vi "Vision Processing.vi"(4 "error in (no error)":errorcluster, 6 "CameraDevRef":T1) -> ()   [LabVIEW 2011]
uses:
  <vilib>/Rock Robotics/WPI/Camera/WPI_CameraDevRef.ctl
  Robot Global Data.vi
  <vilib>/vision/NI_Vision_Development_Module.lvlib
panel:
  out "Aspect Ratio":dbl[](array[numeric])
  out "Offset":dbl
  in  "Max Distance for 1 hoop":dbl=8.0
  out "Raw Turret":dbl
  in  "Run Calculations":bool
  out "Target X Coord":dbl
  out "Target Distance":dbl
  out "Target Y Coord":dbl
  out "Distance Array":dbl[](array[numeric])
  in  "Scaler":dbl=0.85
  in  "Dead Band":dbl=0.05
  out "Number of Rectangles Visible":dbl
  out "Y Position Array":dbl[](array[numeric])
  out "X Position Array":dbl[](array[numeric])
  in  "View":bool
  out "Target Info":T2(array[cluster])
  in  "Area Size Limit":i32=444
  in  "Particle Count Limit":i32=8
  in  "Score Limits":T3={"Rect Coverage"=76.0, "Aspect Ratio"=40.0, "X Edge Strength"=40.0, "Y Edge Strength"=60.0}
  in  "Processing":enum32{"Color", "Intensity", "Intensity Open"}(tab)=enum."Intensity"
  in  "Luminance":i32=255
  in  "Saturation":i32=255
  in  "Hue":i32(knob)=65 scale=0.0..255.0
  in  "Margins":cluster{"Hue":i32, "Sat":i32, "Lum":i32}={"Hue"=20, "Sat"=27, "Lum"=30} {"Sat" scale=0.0..40.0; "Lum" scale=0.0..40.0; "Hue" scale=0.0..40.0}
  in  "Range":cluster{"Lower value":sgl, "Upper value":sgl}={"Lower value"=107.17391, "Upper value"=255.0} {"Lower value" scale=0.0..255.0; "Upper value" scale=0.0..255.0}
  in  "Range":cluster{"Lower value":sgl, "Upper value":sgl}={"Lower value"=123.804344, "Upper value"=255.0} {"Lower value" scale=0.0..255.0; "Upper value" scale=0.0..255.0}
  in  "View":bool
  out "Processed Image":T4(plugin-control)
  out "Original Image":T4(plugin-control)
  # "Instructions:\nProcessing the reflective tape that is illuminated by a ring light can be based\non color or light intensity.\nParticles within the image are scored by rectangle coverage, aspect ratio, and\nfor being hollow with a bold edge. A particle is considered a target if all scores\nare above the score limits. Particles can be annotated -- surrounded by\na rectangle and scores drawn to the left .\nTo control the number of particles being scored, use the count limit and the size\nlimit."
  # "(in)"
  # "To debug, Enable using the View button.\nFor color processing, you can click in the image to select the color for processing."
  # "Enable by clicking the View button.\nGreen scores are above the limit, orange are below. Inner/outer rect\nindicates all passed."
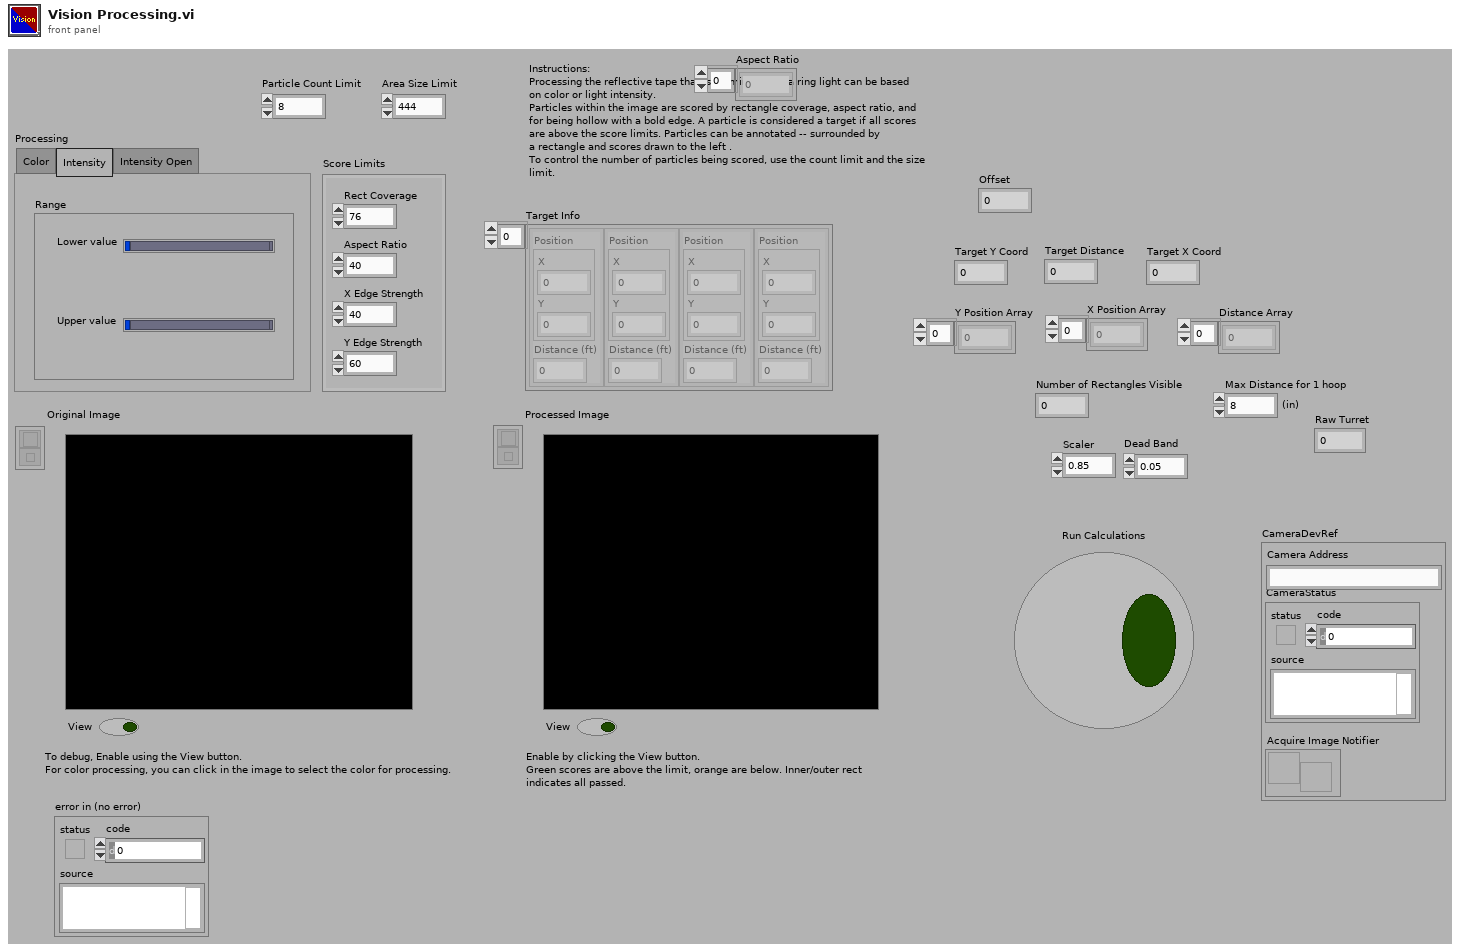
[diagram p1: front panel]
types:
  T1 = typedef "WPI_CameraDevRef.ctl" = cluster{"Camera Address":string, "CameraStatus":errorcluster, "Acquire Image Notifier":refnum<notifier>}
  T2 = cluster{"Position":cluster{"X":dbl, "Y":dbl}, "Distance (ft)":dbl}[]
  T3 = cluster{"Rect Coverage":dbl, "Aspect Ratio":dbl, "X Edge Strength":dbl, "Y Edge Strength":dbl}
  T4 = typedef "IMAQ Image.ctl" = refnum<image>
  T5 = typedef "Image Type" = u32
  T6 = enum32{"AutoM", "Close", "Dilate", "Erode", "Gradient", "Gradient out", "Gradient in", "Hit miss", "Open", "PClose", "POpen", "Thick", "Thin"}
  T7 = typedef "WPI_CameraImageSize.ctl" = enum16{"640x480", "320x240", "160x120"}
  T8 = cluster{"fps":i32, "compression":i32, "Image Size":T7}
  T9 = cluster{cluster{"Left":dbl, "Top":dbl, "Right":dbl, "Bottom":dbl}, dbl[]}[]
  T10 = cluster{"Left":dbl, "Top":dbl, "Right":dbl, "Bottom":dbl}
  T11 = cluster{"Target Center (-1 to 1)":cluster{"X":dbl, "Y":dbl}, "Distance (ft)":dbl}
  T12 = cluster{"Target Center (-1 to 1)":cluster{"X":dbl, "Y":dbl}, "Distance (ft)":dbl}[]
  T13 = typedef "WPI_JoystickDevRef.ctl" = cluster{"Device":T14}
  T14 = typedef "WPI_JoystickDeviceEnum.ctl" = enum16{"USB 1", "USB 2", "USB 3", "USB 4", "Kinect 1", "Kinect 2"}
  T15 = typedef "WPI_JoystickButtonState.ctl" = cluster{"Button 1":bool, "Button 2":bool, "Button 3":bool, "Button 4":bool, "Button 5":bool, "Button 6":bool, "Button 7":bool, "Button 8":bool, "Button 9":bool, "Button 10":bool, "Button 11":bool, "Button 12":bool}
  T16 = cluster{"axis 1 (x)":dbl, "axis 2 (y)":dbl, "axis 3 (throttle)":dbl, "axis 4":dbl, "axis 5":dbl, "axis 6":dbl}
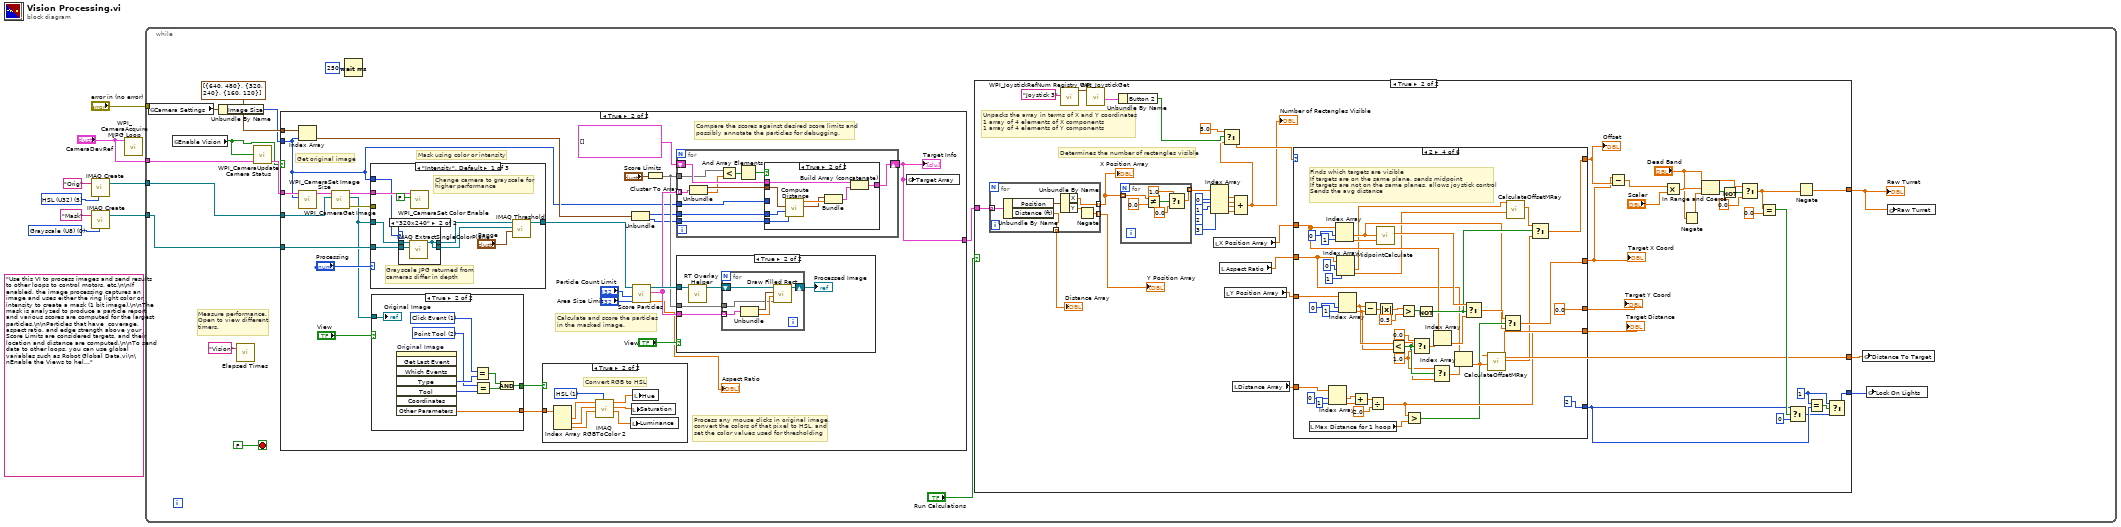
[diagram p0: block diagram]
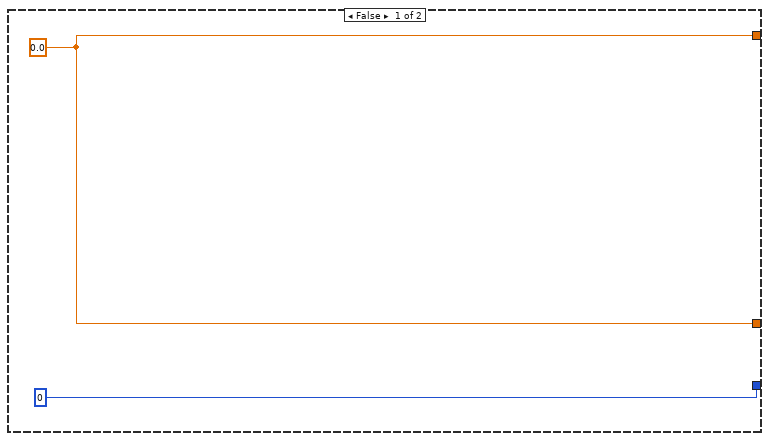
[diagram p2: hidden frame]
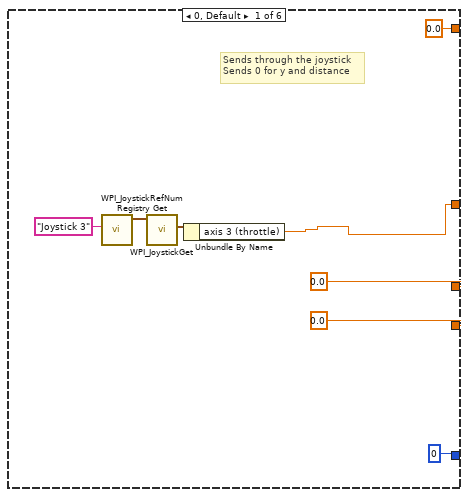
[diagram p3: hidden frame]
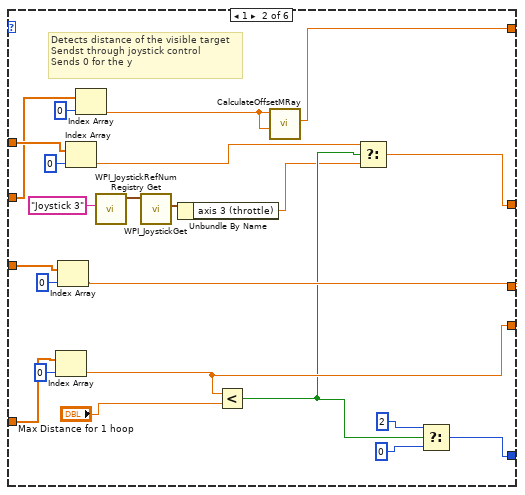
[diagram p4: hidden frame]
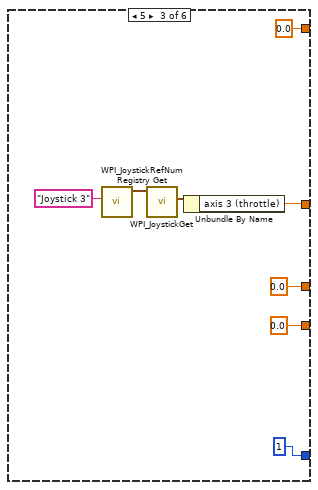
[diagram p5: hidden frame]
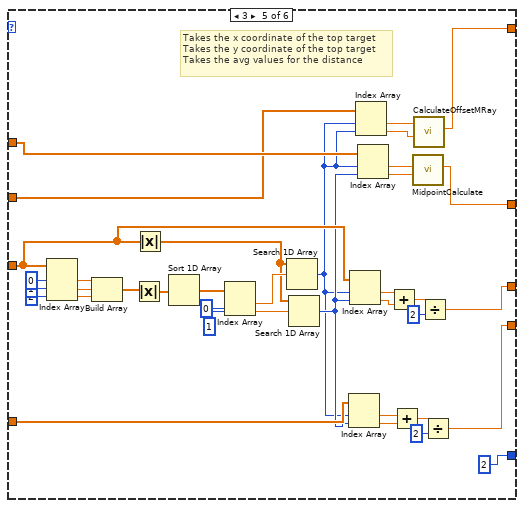
[diagram p6: hidden frame]
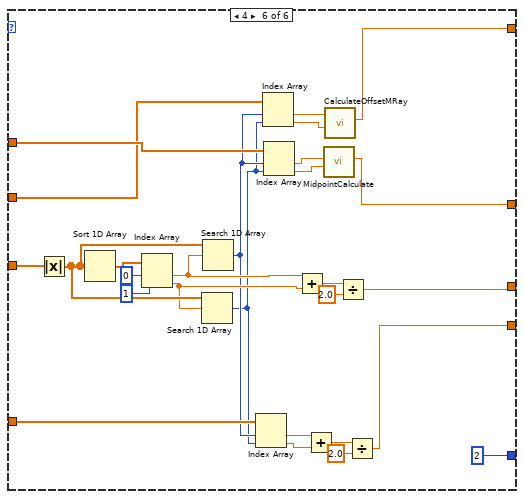
[diagram p7: hidden frame]
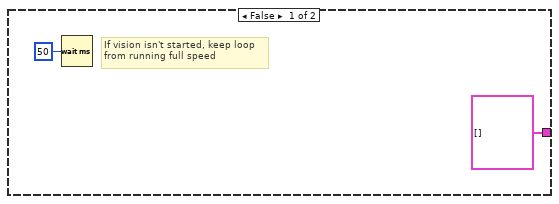
[diagram p8: hidden frame]
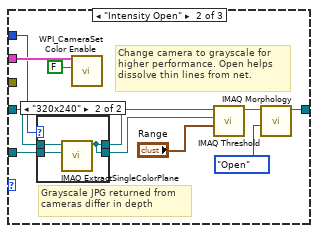
[diagram p11: hidden frame]
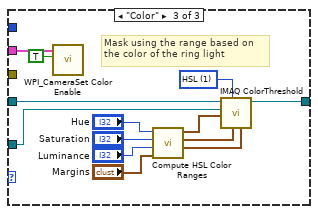
[diagram p13: hidden frame]
diagram:
  w3 = T5 0 items=["Grayscale (U8)", "Grayscale (I16)", "Grayscale (SGL)", "Complex (CSG)", "RGB (U32)", "HSL (U32)", "RGB (U64)", "Grayscale (U16)"] ("Image Type")
  (unwired) "Use this VI to process images and send results to other loops to control motors, etc.\n\nIf enabled, the image processing captures an image and uses either the ring light color or intensity to create a mask (1 bit image).\n\nThe mask is analyzed to produce a particle report and various scores are computed for the largest particles.\n\nParticles that have  coverage, aspect ratio, and edge strength above your Score Limits are considered targets, and their location and distance are computed.\n\nTo send data to other loops, you can use global variables such as Robot Global Data.vi\n\nEnable the Views to help debug color settings. Disable the View to speed up processing."
  w7 = T5 5 items=["Grayscale (U8)", "Grayscale (I16)", "Grayscale (SGL)", "Complex (CSG)", "RGB (U32)", "HSL (U32)", "RGB (U64)", "Grayscale (U16)"] ("Image Type")
  n1 = call "IMAQ Create"("Image Name"="Orig", "Image Type"=w7) -> ("New Image"=w6:T4)  [unwired: 2 in, 2 out]
  n2 = call "IMAQ Create"("Image Name"="Mask", "Image Type"=w3) -> ("New Image"=w1:T4)  [unwired: 2 in, 2 out]
  n3 = call <vilib>:"WPI_CameraAcquire MJPG Loop.vi"("CameraDevRef"="CameraDevRef") -> ()  [unwired: 11 in]
  n4 = while {
    tunnel: w6 -> [w23]
    tunnel: "CameraDevRef" -> [w22]
    tunnel: "error in (no error)" -> [_]
    tunnel: w1 -> [w18]
    stop <- FALSE stop-if-true
    # "Measure performance.\nOpen to view different\ntimers."
    n5 = global read "Robot Global Data.vi" "Camera Settings"() -> (w16:T8)
    n6 = global read "Robot Global Data.vi" "Enable Vision"() -> (w20:bool)
    n7 = Unbundle By Name(w16) -> ("Image Size"=w15:T7)
    n8 = call "Elapsed Times.vi"("Call Name"="Vision") -> ()  [unwired: 2 in, 1 out]
    n9 = call <vilib>:"WPI_CameraUpdate Camera Status.vi"("CameraDevRef In"=w22, "Enable Vision"=w20) -> ("CameraDevRef Out"=w21:T1)  [unwired: 3 in]
    n10 = case shown="True" w20 {
      tunnel: w23 -> [_ w252]
      tunnel: w21 -> [_ w248]
      tunnel: w18 -> [_ w239]
      tunnel: cluster{i32, i32}[] [{640, 480}, {320, 240}, {160, 120}] -> [_ w243]
      tunnel: w15 -> [_ w236]
      tunnel: [T2 [] w237] -> w14
      frame False {
        # "If vision isn't started, keep loop\nfrom running full speed"
        n11 = Wait (ms)(milliseconds to wait=u32 50) -> ()  [unwired: 1 out]
      }
      frame True {
        # "Compare the scores against desired score limits and\npossibly annotate the particles for debugging."
        # "Process any mouse clicks in original image,\nconvert the colors of that pixel to HSL, and\nset the color values used for thresholding"
        # "Calculate and score the particles\nin the masked image."
        # "Mask using color or intensity"
        # "Get original image"
        n12 = call <vilib>:"WPI_CameraSet Image Size.vi"("Image Size"=w236, "CameraDevRef"=w248) -> ("CameraDevRef Out"=w249:T1)  [unwired: 8 in, 1 out]
        n13 = Index Array(array=w243, index=w236) -> (element=w240:cluster{i32, i32})
        n14 = call <vilib>:"WPI_CameraGet Image.vi"("Image"=w252, "CameraDevRef"=w249) -> ("error out"=w250:errorcluster, "Image Out"=w238:T4, "CameraDevRef Out"=w251:T1)  [unwired: 7 in]
        n15 = case shown="\"Intensity\", Default" "Processing" {
          tunnel: w238 -> [w274 w286 w312]
          tunnel: [w277 w291 w311] -> w246
          tunnel: w251 -> [w275 w289 w302]
          tunnel: w250 -> [_ _ _]
          tunnel: w239 -> [w273 w287 w300]
          tunnel: w236 -> [w272 w288 _]
          frame "Intensity", Default {
            # "Grayscale JPG returned from\ncameras differ in depth"
            # "Change camera to grayscale for\nhigher performance"
            n16 = case shown="\"320x240\"" w272 {
              tunnel: w274 -> [w280 w283]
              tunnel: w273 -> [w279 w282]
              tunnel: [w280 w281] -> w271
              tunnel: [w279 w281] -> w270
              frame "640x480", Default {
              }
              frame "320x240" {
                n17 = call "IMAQ ExtractSingleColorPlane"("Image Dst"=w282, "Image Src"=w283) -> ("Image Dst Out"=w281:T4)  [unwired: 8 in, 1 out]
              }
            }
            n18 = call <vilib>:"WPI_CameraSet Color Enable.vi"("Color Enabled"=FALSE, "CameraDevRef"=w275) -> ()  [unwired: 8 in, 2 out]
            n19 = call "IMAQ Threshold"("Range"="Range", "Image Dst"=w270, "Image Src"=w271) -> ("Image Dst Out"=w277:T4)  [unwired: 3 in, 5 out]
          }
          frame "Intensity Open" {
            # "Grayscale JPG returned from\ncameras differ in depth"
            # "Change camera to grayscale for\nhigher performance. Open helps\ndissolve thin lines from net."
            n20 = case shown="\"320x240\"" w288 {
              tunnel: w286 -> [w296 w299]
              tunnel: w287 -> [w295 w298]
              tunnel: [w296 w297] -> w285
              tunnel: [w295 w297] -> w284
              frame "640x480", Default {
              }
              frame "320x240" {
                n21 = call "IMAQ ExtractSingleColorPlane"("Image Dst"=w298, "Image Src"=w299) -> ("Image Dst Out"=w297:T4)  [unwired: 8 in, 1 out]
              }
            }
            n22 = call <vilib>:"WPI_CameraSet Color Enable.vi"("Color Enabled"=FALSE, "CameraDevRef"=w289) -> ()  [unwired: 8 in, 2 out]
            n23 = call "IMAQ Threshold"("Range"="Range", "Image Dst"=w284, "Image Src"=w285) -> ("Image Dst Out"=w292:T4)  [unwired: 3 in, 5 out]
            n24 = call "IMAQ Morphology"("Operation"=T6."Open", "Image Src"=w292) -> ("Image Dst Out"=w291:T4)  [unwired: 8 in, 1 out]
          }
          frame "Color" {
            w310 = u16 1 items=["RGB", "HSL", "HSV", "HSI"] ("Color Mode")
            # "Mask using the range based on\nthe color of the ring light"
            n25 = call <vilib>:"WPI_CameraSet Color Enable.vi"("Color Enabled"=TRUE, "CameraDevRef"=w302) -> ()  [unwired: 8 in, 2 out]
            n26 = call "Compute HSL Color Ranges.vi"("Margins"="Margins", "Luminance"="Luminance", "Saturation"="Saturation", "Hue"="Hue") -> ("Lum Range"=w307:cluster{i32, i32}, "Sat Range"=w308:cluster{i32, i32}, "Hue Range"=w309:cluster{i32, i32})  [unwired: 5 in]
            n27 = call "IMAQ ColorThreshold"("Blue or Luma or Val or Inten Range"=w307, "Green or Sat Range"=w308, "Color Mode"=w310, "Red or Hue Range"=w309, "Image Dst"=w300, "Image Src"=w312) -> ("Image Dst Out"=w311:T4)  [unwired: 4 in, 1 out]
          }
        }
        n28 = case shown="True" "View" {
          tunnel: w238 -> [_ w332]
          tunnel: [_ w327] -> w245
          tunnel: [_ w324] -> w244
          frame False {
          }
          frame True {
            w325 = 2 items=["None", "Selection Tool", "Point Tool", "Line Tool", "Rectangle Tool", "Oval Tool", "Polygon Tool", "ClosedFreehandTool", "Annulus Tool", "Rotated Rectangle Tool", "Zoom Tool", "Pan Tool", "Polyline Tool", "Freehand Tool"] ("Tool")
            w326 = 1 items=["No Event"=0, "Click Event"=1, "Draw Event"=2, "Size Event"=4, "Scroll Event"=5, "Double Click Event"=8] ("Type")
            n29 = invoke on="Original Image" class="ImageControl" method="Get Last Event"() -> ("Type"=w328:i32, "Tool"=w331:i32, "Other Parameters"=w324:sgl[])  [unwired: 8 in, 5 out]
            n30 = Equal?(x=w326, y=w328) -> (x = y?=w329:bool)
            n31 = Equal?(x=w325, y=w331) -> (x = y?=w330:bool)
            n32 = And(x=w329, y=w330) -> (x .and. y?=w327:bool)
            "Original Image" <- w332
          }
        }
        n33 = case shown="True" w245 {
          tunnel: w244 -> [_ w269]
          frame False {
          }
          frame True {
            w268 = u16 1 items=["RGB", "HSL", "HSV", "HSI", "CIE L*a*b*", "CIE XYZ"] ("Color Mode")
            # "Convert RGB to HSL"
            n34 = Index Array(array=w269) -> (element #1=w267:sgl, element #2=w265:sgl, element #3=w263:sgl)  [unwired: 3 in]
            n35 = call "IMAQ RGBToColor 2"("Color Mode"=w268, "Blue value"=w263, "Green value"=w265, "Red value"=w267) -> ("Blue or Luma or Val or Inten or Z or b*value"=w262:dbl, "Green or Sat or Y or a* value"=w264:dbl, "Red or Hue or X or L* value"=w266:dbl)  [unwired: 4 in, 1 out]
            n36 = local write "Luminance"(w262) -> ()
            n37 = local write "Saturation"(w264) -> ()
            n38 = local write "Hue"(w266) -> ()
          }
        }
        n39 = Unbundle(w240) -> (w242:i32, w241:i32)
        n40 = call "Score Particles.vi"("Area Size Limit"="Area Size Limit", "Particle Count Limit"="Particle Count Limit", "Image Refnum in"=w246) -> ("Aspect Ratio"=→"Aspect Ratio":dbl[], "Scored Particle Info"=w257:T9, "Image Refnum out"=w260:T4)  [unwired: 6 in]
        n41 = Cluster To Array(cluster="Score Limits") -> (array=w255:dbl[])
        n42 = for {
          shift-right: [w342] -> w237
          shift-left: T2 [] -> [w343]
          tunnel: w242 -> [w341]
          tunnel: w257 -> [w339] mode=indexing
          tunnel: w255 -> [w334]
          tunnel: w236 -> [w338]
          tunnel: w241 -> [w333]
          n43 = Unbundle(w339) -> (w340:T10, w335:dbl[])
          n44 = Less?(x=w334, y=w335) -> (x < y?=w337:bool[])
          n45 = And Array Elements(Boolean array=w337) -> (logical AND=w336:bool)
          n46 = case shown="True" w336 {
            tunnel: w343 -> [w344 w352]
            tunnel: [w344 w351] -> w342
            tunnel: w340 -> [_ w347]
            tunnel: w341 -> [_ w349]
            tunnel: w338 -> [_ _]
            tunnel: w333 -> [_ w346]
            frame False {
            }
            frame True {
              n47 = call "Compute Distance.vi"("Y Image Resolution"=w346, "X Image Resolution"=w349, "Bounding Box"=w347) -> ("Target Center (-1 to 1)"=w345:cluster{"X":dbl, "Y":dbl}, "Distance (ft)"=w348:dbl)  [unwired: 7 in]
              n48 = Bundle("Target Center (-1 to 1)"=w345, "Distance (ft)"=w348) -> (w350:T11)  [unwired: 1 in]
              n49 = Build Array (concatenate)(w352, w350) -> (w351:T12)
            }
          }
        }
        "Target Info" <- w237
        n50 = case shown="True" "View" {
          tunnel: w260 -> [_ w314]
          tunnel: w257 -> [_ w316]
          tunnel: w255 -> [_ w315]
          frame False {
          }
          frame True {
            n51 = call "RT Overlay Helper.vi"("Refnum in"=w314) -> ("Refnum out"=w317:T4)  [unwired: 10 in]
            n52 = for {
              shift-right: [w322] -> w313
              shift-left: w317 -> [w323]
              tunnel: w316 -> [w319] mode=indexing
              tunnel: w315 -> [w318]
              n53 = Unbundle(w319) -> (w320:T10, w321:dbl[])
              n54 = call "Draw Filled Rect.vi"("Limits"=w318, "Scores"=w321, "Bounding Box"=w320, "image in"=w323) -> ("image out"=w322:T4)  [unwired: 7 in]
            }
            "Processed Image" <- w313
          }
        }
        n55 = global write "Robot Global Data.vi" "Target Array"(w237) -> ()
      }
    }
    n56 = Wait (ms)(milliseconds to wait=u32 250) -> ()  [unwired: 1 out]
    n57 = case shown="True" "Run Calculations" {
      tunnel: w14 -> [_ w48]
      tunnel: [w25 w32] -> w11
      tunnel: [0 ("f") w40] -> w10
      tunnel: [w25 w35] -> w9
      frame False {
        w25 = 0.0 ("f")
      }
      frame True {
        w41 = 1 ("y")
        # "Determines the number of rectangles visible"
        # "Unpacks the array in terms of X and Y coordinates\n1 array of 4 elements of X components\n1 array of 4 elements of Y components"
        n58 = for {
          tunnel: [w230] -> w49 mode=indexing
          tunnel: [w231] -> w59 mode=indexing
          tunnel: w48 -> [w228] mode=indexing
          tunnel: [w227] -> w67 mode=indexing
          n59 = Unbundle By Name(w228) -> ("Position"=w232:cluster{"X":dbl, "Y":dbl}, "Distance (ft)"=w227:dbl)
          n60 = Unbundle By Name(w232) -> ("X"=w231:dbl, "Y"=w229:dbl)
          n61 = Negate(x=w229) -> (-x=w230:dbl)
        }
        "X Position Array" <- w59
        "Y Position Array" <- w49
        "Distance Array" <- w67
        n62 = call <vilib>:"WPI_JoystickRefNum Registry Get.vi"("refnum name"="Joystick 3") -> ("JoystickDevRef"=w46:T13)  [unwired: 9 in, 1 out]
        n63 = call <vilib>:"WPI_JoystickGet.vi"("JoystickDevRef"=w46) -> ("Buttons"=w44:T15)  [unwired: 4 in, 2 out]
        n64 = Unbundle By Name(w44) -> ("Button 2"=w43:bool)
        n65 = for {
          tunnel: w59 -> [w77] mode=indexing
          tunnel: [w73] -> w58 mode=indexing
          n66 = Not Equal?(x=w77, y=0.0) -> (x != y?=w76:bool)
          n67 = Select(t=1.0, s=w76, f=0.0) -> (s? t:f=w73:dbl)
        }
        n68 = Index Array(array=w58, index #1=0 ("index"), index #2=1 ("index"), index #3=2 ("index"), index #4=3 ("index")) -> (element #1=w56:dbl, element #2=w57:dbl, element #3=w55:dbl, element #4=w54:dbl)
        n69 = local read "X Position Array"() -> (w60:dbl[])
        n70 = local read "Aspect Ratio"() -> (w31:dbl[])
        n71 = local read "Y Position Array"() -> (w69:dbl[])
        n72 = local read "Distance Array"() -> (w70:dbl[])
        n73 = Compound Arithmetic op=ADD(w56, w57, w55, w54) -> (w34:dbl)
        "Number of Rectangles Visible" <- w34
        n74 = Select(t=5.0, s=w43, f=w34) -> (s? t:f=w71:dbl)
        n75 = case shown="2" w71 {
          tunnel: w60 -> [_ w106 _ w126 w183 w221]
          tunnel: [w80 w100 w111 w136 w182 w215] -> w29
          tunnel: [0.0 ("X") w97 0.0 ("X") 0.0 ("X") w184 w214] -> w68
          tunnel: [0.0 ("X") w102 0.0 ("X") w139 w171 w209] -> w35
          tunnel: w69 -> [_ w98 _ w160 w178 w226]
          tunnel: w70 -> [_ w109 _ w148 w173 w220]
          tunnel: [0 w93 1 2 2 2] -> w38
          tunnel: [0.0 ("Offset") w90 0.0 ("Offset") w123 w167 w205] -> w30
          tunnel: w31 -> [_ w89 _ w118 w163 w200]
          frame 0, Default {
            # "Sends through the joystick\nSends 0 for y and distance"
            n76 = call <vilib>:"WPI_JoystickRefNum Registry Get.vi"("refnum name"="Joystick 3") -> ("JoystickDevRef"=w84:T13)  [unwired: 9 in, 1 out]
            n77 = call <vilib>:"WPI_JoystickGet.vi"("JoystickDevRef"=w84) -> ("Axes"=w82:T16)  [unwired: 4 in, 2 out]
            n78 = Unbundle By Name(w82) -> ("axis 3 (throttle)"=w80:dbl)
          }
          frame 1 {
            # "Detects distance of the visible target\nSendst through joystick control\nSends 0 for the y"
            n79 = Index Array(array=w109, index=0) -> (element=w102:dbl)
            n80 = Index Array(array=w98, index=0) -> (element=w97:dbl)
            n81 = Index Array(array=w106, index=0) -> (element=w91:dbl)
            n82 = Index Array(array=w89, index=0) -> (element=w87:dbl)
            n83 = call <vilib>:"WPI_JoystickRefNum Registry Get.vi"("refnum name"="Joystick 3") -> ("JoystickDevRef"=w105:T13)  [unwired: 9 in, 1 out]
            n84 = call <vilib>:"WPI_JoystickGet.vi"("JoystickDevRef"=w105) -> ("Axes"=w103:T16)  [unwired: 4 in, 2 out]
            n85 = Unbundle By Name(w103) -> ("axis 3 (throttle)"=w92:dbl)
            n86 = Less?(x=w102, y="Max Distance for 1 hoop") -> (x < y?=w95:bool)
            n87 = call "CalculateOffsetMRay.vi"("AR2"=w87, "AR1"=w87) -> ("Offset"=w90:dbl)  [unwired: 9 in]
            n88 = Select(t=w91, s=w95, f=w92) -> (s? t:f=w100:dbl)
            n89 = Select(t=2, s=w95, f=0) -> (s? t:f=w93:i32)
          }
          frame 5 {
            n90 = call <vilib>:"WPI_JoystickRefNum Registry Get.vi"("refnum name"="Joystick 3") -> ("JoystickDevRef"=w115:T13)  [unwired: 9 in, 1 out]
            n91 = call <vilib>:"WPI_JoystickGet.vi"("JoystickDevRef"=w115) -> ("Axes"=w113:T16)  [unwired: 4 in, 2 out]
            n92 = Unbundle By Name(w113) -> ("axis 3 (throttle)"=w111:dbl)
          }
          frame 2 {
            w129 = 1.0 ("f")
            w128 = 0.0 ("t")
            # "Finds which targets are visible\nIf targets are on the same plane, sends midpoint\nIf targets are not on the same planes, allows joystick control\nSends the avg distance"
            n93 = local read "Max Distance for 1 hoop"() -> (w138:dbl)
            n94 = Index Array(array=w148, index #1=0 ("index"), index #2=1 ("index")) -> (element #1=w147:dbl, element #2=w146:dbl)
            n95 = Index Array(array=w126, index #1=0 ("index"), index #2=1 ("index")) -> (element #1=w133:dbl, element #2=w132:dbl)
            n96 = Index Array(array=w118, index #1=0 ("index"), index #2=1 ("index")) -> (element #1=w120:dbl, element #2=w119:dbl)
            n97 = Index Array(array=w160, index #1=0 ("index"), index #2=1 ("index")) -> (element #1=w144:dbl, element #2=w143:dbl)
            n98 = Add(x=w147, y=w146) -> (x+y=w151:dbl)
            n99 = Subtract(x=w144, y=w143) -> (x-y=w157:dbl)
            n100 = Divide(x=w151, y=2.0) -> (x/y=w139:dbl)
            n101 = call "MidpointCalculate.vi"("X2"=w132, "X1"=w133) -> ("Midpoint"=w153:dbl)  [unwired: 9 in]
            n102 = Absolute Value(x=w157) -> (abs(x)=w156:dbl)
            n103 = Less?(x=w144, y=w143) -> (x < y?=w130:bool)
            n104 = Greater?(x=w156, y=0.5) -> (0:w154:bool)
            n105 = Greater?(x=w139, y=w138) -> (0:w137:bool)
            n106 = Select(t=w128, s=w130, f=w129) -> (s? t:f=w142:dbl)
            n107 = Not(x=w154) -> (.not. x?=w134:bool)
            n108 = Select(t=w129, s=w130, f=w128) -> (s? t:f=w127:dbl)
            n109 = Index Array(array=w126, index=w142) -> (element=w141:dbl)
            n110 = Index Array(array=w118, index=w127) -> (element=w125:dbl)
            n111 = Select(t=w153, s=w134, f=w141) -> (s? t:f=w135:dbl)
            n112 = call "CalculateOffsetMRay.vi"("AR2"=w125, "AR1"=w125) -> ("Offset"=w124:dbl)  [unwired: 9 in]
            n113 = Select(t=w135, s=w137, f=w133) -> (s? t:f=w136:dbl)
            n114 = call "CalculateOffsetMRay.vi"("AR2"=w119, "AR1"=w120) -> ("Offset"=w131:dbl)  [unwired: 9 in]
            n115 = Select(t=w131, s=w134, f=w124) -> (s? t:f=w123:dbl)
          }
          frame 3 {
            # "Takes the x coordinate of the top target\nTakes the y coordinate of the top target\nTakes the avg values for the distance"
            n116 = Index Array(array=w178, index #1=0 ("index"), index #2=1 ("index"), index #3=2 ("index")) -> (element #1=w196:dbl, element #2=w195:dbl, element #3=w194:dbl)
            n117 = Build Array(w196, w195, w194) -> (w193:dbl[])
            n118 = Absolute Value(x=w193) -> (abs(x)=w187:dbl[])
            n119 = Absolute Value(x=w178) -> (abs(x)=w181:dbl[])
            n120 = Sort 1D Array(array=w187) -> (sorted array=w192:dbl[])
            n121 = Index Array(array=w192, index #1=0 ("index"), index #2=1 ("index")) -> (element #1=w188:dbl, element #2=w189:dbl)
            n122 = Search 1D Array(1D array=w181, element=w188) -> (index of element=w166:i32)  [unwired: 1 in]
            n123 = Search 1D Array(1D array=w181, element=w189) -> (index of element=w172:i32)  [unwired: 1 in]
            n124 = Index Array(array=w173, index #1=w166, index #2=w172) -> (element #1=w175:dbl, element #2=w174:dbl)
            n125 = Index Array(array=w178, index #1=w166, index #2=w172) -> (element #1=w180:dbl, element #2=w179:dbl)
            n126 = Index Array(array=w163, index #1=w166, index #2=w166) -> (element #1=w165:dbl, element #2=w164:dbl)
            n127 = Index Array(array=w183, index #1=w166, index #2=w172) -> (element #1=w169:dbl, element #2=w168:dbl)
            n128 = Add(x=w180, y=w179) -> (x+y=w186:dbl)
            n129 = Add(x=w175, y=w174) -> (x+y=w176:dbl)
            n130 = call "MidpointCalculate.vi"("X2"=w168, "X1"=w169) -> ("Midpoint"=w182:dbl)  [unwired: 9 in]
            n131 = call "CalculateOffsetMRay.vi"("AR2"=w164, "AR1"=w165) -> ("Offset"=w167:dbl)  [unwired: 9 in]
            n132 = Divide(x=w186, y=2) -> (x/y=w184:dbl)
            n133 = Divide(x=w176, y=2) -> (x/y=w171:dbl)
          }
          frame 4 {
            n134 = Absolute Value(x=w226) -> (abs(x)=w222:dbl[])
            n135 = Sort 1D Array(array=w222) -> (sorted array=w225:dbl[])
            n136 = Index Array(array=w225, index #1=0 ("index"), index #2=1 ("index")) -> (element #1=w219:dbl, element #2=w218:dbl)
            n137 = Search 1D Array(1D array=w222, element=w218) -> (index of element=w203:i32)  [unwired: 1 in]
            n138 = Search 1D Array(1D array=w222, element=w219) -> (index of element=w204:i32)  [unwired: 1 in]
            n139 = Index Array(array=w220, index #1=w204, index #2=w203) -> (element #1=w211:dbl, element #2=w210:dbl)
            n140 = Index Array(array=w200, index #1=w204, index #2=w203) -> (element #1=w201:dbl, element #2=w202:dbl)
            n141 = Index Array(array=w221, index #1=w204, index #2=w203) -> (element #1=w207:dbl, element #2=w206:dbl)
            n142 = Add(x=w219, y=w218) -> (x+y=w217:dbl)
            n143 = Add(x=w211, y=w210) -> (x+y=w212:dbl)
            n144 = call "MidpointCalculate.vi"("X2"=w206, "X1"=w207) -> ("Midpoint"=w215:dbl)  [unwired: 9 in]
            n145 = call "CalculateOffsetMRay.vi"("AR2"=w202, "AR1"=w201) -> ("Offset"=w205:dbl)  [unwired: 9 in]
            n146 = Divide(x=w217, y=2.0) -> (x/y=w214:dbl)
            n147 = Divide(x=w212, y=2.0) -> (x/y=w209:dbl)
          }
        }
        "Target Y Coord" <- w68
        "Target Distance" <- w35
        "Target X Coord" <- w29
        "Offset" <- w30
        n148 = Subtract(x=w29, y=w30) -> (x-y=w28:dbl)
        n149 = Multiply(x=w28, y="Scaler") -> (x*y=w66:dbl)
        n150 = Negate(x="Dead Band") -> (-x=w62:dbl)
        n151 = In Range and Coerce(upper limit="Dead Band", x=w66, lower limit=w62) -> (In Range?=w63:bool)  [unwired: 1 out]
        n152 = Not(x=w63) -> (.not. x?=w64:bool)
        n153 = Select(t=w66, s=w64, f=0.0) -> (s? t:f=w33:dbl)
        n154 = Equal?(x=w33, y=0.0) -> (x = y?=w39:bool)
        n155 = Select(t=w38, s=w39, f=0) -> (s? t:f=w36:i32)
        n156 = Negate(x=w33) -> (-x=w32:dbl)
        n157 = Equal?(x=w41, y=w38) -> (x = y?=w42:bool)
        n158 = Select(t=w41, s=w42, f=w36) -> (s? t:f=w40:i32)
      }
    }
    "Raw Turret" <- w11
    n159 = global write "Robot Global Data.vi" "Distance To Target"(w9) -> ()
    n160 = global write "Robot Global Data.vi" "Lock On Lights"(w10) -> ()
    n161 = global write "Robot Global Data.vi" "Raw Turret"(w11) -> ()
  }
